vi "Convert to Pump Interface State.vi"(8 "error in (no error)":errorcluster, 11 "Instrument State in":T2) -> (0 "error out":errorcluster, 3 "Pump State out":variant)   [LabVIEW 2020, in "Mock Pump Controller.lvlib" / "Remote Connection Manager.lvlib"]
uses:
  Remote Connection Manager.lvlib
  Instrument Manager/Instrument State.ctl
  Typedefs/Pump Controller State.ctl
  Mock Pump Controller.lvlib
  Instrument Manager/Instrument Manager.lvlib
panel:
  out "Pump Controller State":T1
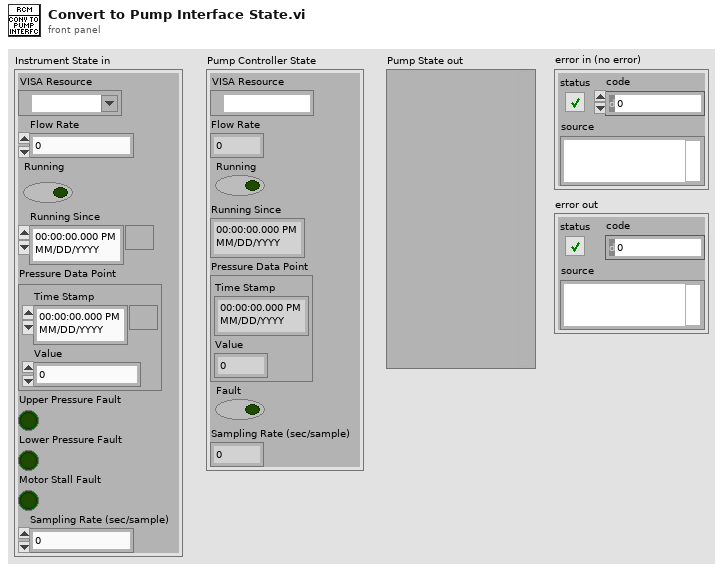
[diagram p1: front panel]
types:
  T1 = typedef "Mock Pump Controller.lvlib/Pump Controller State.ctl" = cluster{"VISA Resource":refnum<visa-resource-name>, "Flow Rate":dbl, "Running":bool, "Running Since":timestamp, "Pressure Data Point":cluster{"Time Stamp":timestamp, "Value":dbl}, "Fault":bool, "Sampling Rate (sec/sample)":dbl}
  T2 = typedef "Mock Pump Controller.lvlib/Instrument Manager.lvlib/Instrument State.ctl" = cluster{"VISA Resource":refnum<visa-resource-name>, "Flow Rate":dbl, "Running":bool, "Running Since":timestamp, "Pressure Data Point":cluster{"Time Stamp":timestamp, "Value":dbl}, "Upper Pressure Fault":bool, "Lower Pressure Fault":bool, "Motor Stall Fault":bool, "Sampling Rate (sec/sample)":dbl}
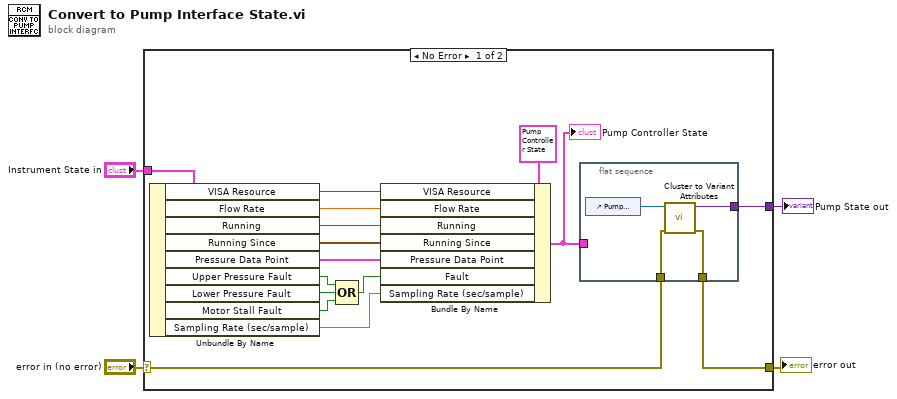
[diagram p0: block diagram]
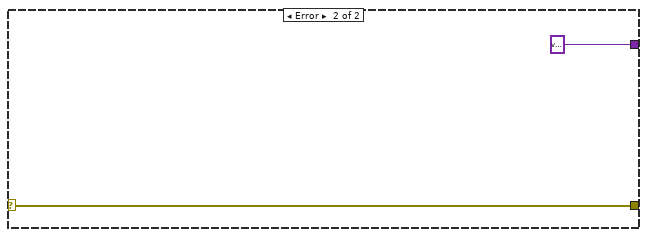
[diagram p2: hidden frame]
diagram:
  n1 = case shown="No Error" "error in (no error)" {
    selector: "error in (no error)" -> [w8 w26]
    tunnel: "Instrument State in" -> [w20 _]
    tunnel: [w7 w26] -> w2
    tunnel: [w5 variant] -> w1
    frame No Error {
      n2 = Unbundle By Name(w20) -> ("VISA Resource"=w19:refnum<visa-resource-name>, "Flow Rate"=w18:dbl, "Running"=w17:bool, "Running Since"=w16:timestamp, "Pressure Data Point"=w15:cluster{"Time Stamp":timestamp, "Value":dbl}, "Upper Pressure Fault"=w14:bool, "Lower Pressure Fault"=w13:bool, "Motor Stall Fault"=w12:bool, "Sampling Rate (sec/sample)"=w10:dbl)
      n3 = Compound Arithmetic op=OR(w14, w13, w12) -> (w11:bool)
      n4 = Bundle By Name(cluster=T1 {"VISA Resource"="", "Flow Rate"=0.0, "Running"=FALSE, "Running Since"=timestamp(0 s since 1904-01-01), "Pressure Data Point"={"Time Stamp"=timestamp(0 s since 1904-01-01), "Value"=0.0}, "Fault"=FALSE, "Sampling Rate (sec/sample)"=0.0} ("Pump Controller State"), "VISA Resource"=w19, "Flow Rate"=w18, "Running"=w17, "Running Since"=w16, "Pressure Data Point"=w15, "Fault"=w11, "Sampling Rate (sec/sample)"=w10) -> (w6:T1)
      "Pump Controller State" <- w6
      n5 = flat-sequence {
        tunnel: w8 -> [w23]
        tunnel: [w22] -> w7
        tunnel: w6 -> [_]
        tunnel: [w21] -> w5
        frame #0 {
          n6 = control-ref of="Pump Controller State"() -> (w24:refnum<vi>)
          n7 = call "Cluster to Variant Attributes.vi"("error in (no error)"=w23, "Cluster in"=w24) -> ("error out"=w22:errorcluster, "Variant out"=w21:variant)  [unwired: 8 in]
        }
      }
    }
    frame Error {
    }
  }
  "error out" <- w2
  "Pump State out" <- w1
